vi "rsscope_core_global.vi"() -> ()   [LabVIEW 2018] (continued)
MIL1553 trigger word count/ mode code settings."}, {"Level"=5, "Class Only"=FALSE, "Identifier"="RSSCOPE_ATTR_PROTOCOL_MIL1553_TRIGGER_WORD_COUNT_PATTERN_CONDITION", "Descriptive Name"="Protocol MIL1553 Trigger Word Count Pattern Condition", "Data Type"=0, "Command"="TRIG{Trigger}:MILS:CMD:CCON", "Access"=2, "Range Table"="rsscope_rngProtocolMIL1553WordCountOperator", "Read Callback"="", "Write Callback"="", "Supported Models"="RTO|RTP", "Instrument Options"="", "Flags"=0, "Help"="Sets the operator to set a specific data word count or mode code pattern.\n\nAvailable Repeated Capabilities:\nTrigger: TrigA, TrigB, TrigR\r\n\nRemote-control command(s):\nTRIGger<m>:MILStd:CMD:CCONdition"}, {"Level"=5, "Class Only"=FALSE, "Identifier"="RSSCOPE_ATTR_PROTOCOL_MIL1553_TRIGGER_WORD_COUNT_PATTERN_MIN", "Descriptive Name"="Protocol MIL1553 Trigger Word Count Pattern Min", "Data Type"=2, "Command"="TRIG{Trigger}:MILS:CMD:CMIN", "Access"=2, "Range Table"="", "Read Callback"="", "Write Callback"="", "Supported Models"="RTO|RTP", "Instrument Options"="", "Flags"=0, "Help"="Specifies a data word count/mode code pattern or sets the start value of a pattern range.\n\nAvailable Repeated Capabilities:\nTrigger: TrigA, TrigB, TrigR\r\n\nRemote-control command(s):\nTRIGger<m>:MILStd:CMD:CMIN"}, {"Level"=5, "Class Only"=FALSE, "Identifier"="RSSCOPE_ATTR_PROTOCOL_MIL1553_TRIGGER_WORD_COUNT_PATTERN_MAX", "Descriptive Name"="Protocol MIL1553 Trigger Word Count Pattern Max", "Data Type"=2, "Command"="TRIG{Trigger}:MILS:CMD:CMAX", "Access"=2, "Range Table"="", "Read Callback"="", "Write Callback"="", "Supported Models"="RTO|RTP", "Instrument Options"="", "Flags"=0, "Help"="Sets the end value of a data word count/mode code pattern if &apos;Word Count Condition&apos; is set to InRange or OutOfRange.\n\nAvailable Repeated Capabilities:\nTrigger: TrigA, TrigB, TrigR\r\n\nRemote-control command(s):\nTRIGger<m>:MILStd:CMD:CMAX"}, {"Level"=3, "Class Only"=TRUE, "Identifier"="", "Descriptive Name"="Status Flags", "Data Type"=0, "Command"="", "Access"=0, "Range Table"="", "Read Callback"="", "Write Callback"="", "Supported Models"="", "Instrument Options"="", "Flags"=0, "Help"="Specifies the values of the status flags. You can use the following characters: 1; 0; or X (don&apos;t care)."}, {"Level"=4, "Class Only"=FALSE, "Identifier"="RSSCOPE_ATTR_PROTOCOL_MIL1553_TRIGGER_STATUS_FLAG_MESSAGE_ERROR", "Descriptive Name"="Protocol MIL1553 Trigger Status Flag Message Error", "Data Type"=0, "Command"="TRIG{Trigger}:MILS:STAT:MERR", "Access"=2, "Range Table"="rsscope_rngProtocolMIL1553TriggerStatusFlags", "Read Callback"="", "Write Callback"="", "Supported Models"="RTO|RTP", "Instrument Options"="", "Flags"=0, "Help"="Triggers on the state of the message error bit of the status word if &apos;Trigger Mode&apos; is set to StatusWord.\n\nAvailable Repeated Capabilities:\nTrigger: TrigA, TrigB, TrigR\r\n\nRemote-control command(s):\nTRIGger<m>:MILStd:STATus:MERRor"}, {"Level"=4, "Class Only"=FALSE, "Identifier"="RSSCOPE_ATTR_PROTOCOL_MIL1553_TRIGGER_STATUS_FLAG_BUSY", "Descriptive Name"="Protocol MIL1553 Trigger Status Flag Busy", "Data Type"=0, "Command"="TRIG{Trigger}:MILS:STAT:BUSY", "Access"=2, "Range Table"="rsscope_rngProtocolMIL1553TriggerStatusFlags", "Read Callback"="", "Write Callback"="", "Supported Models"="RTO|RTP", "Instrument Options"="", "Flags"=0, "Help"="Triggers on the state of the busy bit of the status word if &apos;Trigger Mode&apos; is set to StatusWord.\n\nAvailable Repeated Capabilities:\nTrigger: TrigA, TrigB, TrigR\r\n\nRemote-control command(s):\nTRIGger<m>:MILStd:STATus:BUSY"}, {"Level"=4, "Class Only"=FALSE, "Identifier"="RSSCOPE_ATTR_PROTOCOL_MIL1553_TRIGGER_STATUS_FLAG_INSTRUMENTATION", "Descriptive Name"="Protocol MIL1553 Trigger Status Flag Instrumentation", "Data Type"=0, "Command"="TRIG{Trigger}:MILS:STAT:INST", "Access"=2, "Range Table"="rsscope_rngProtocolMIL1553TriggerStatusFlags", "Read Callback"="", "Write Callback"="", "Supported Models"="RTO|RTP", "Instrument Options"="", "Flags"=0, "Help"="Triggers on the state of the instrumentation bit of the status word if &apos;Trigger Mode&apos; is set to StatusWord.\n\nAvailable Repeated Capabilities:\nTrigger: TrigA, TrigB, TrigR\r\n\nRemote-control command(s):\nTRIGger<m>:MILStd:STATus:INSTrument"}, {"Level"=4, "Class Only"=FALSE, "Identifier"="RSSCOPE_ATTR_PROTOCOL_MIL1553_TRIGGER_STATUS_FLAG_SUBSYSTEM", "Descriptive Name"="Protocol MIL1553 Trigger Status Flag Subsystem", "Data Type"=0, "Command"="TRIG{Trigger}:MILS:STAT:SUBS", "Access"=2, "Range Table"="rsscope_rngProtocolMIL1553TriggerStatusFlags", "Read Callback"="", "Write Callback"="", "Supported Models"="RTO|RTP", "Instrument Options"="", "Flags"=0, "Help"="Triggers on the state of the subsystem flag bit of the status word if &apos;Trigger Mode&apos; is set to StatusWord.\n\nAvailable Repeated Capabilities:\nTrigger: TrigA, TrigB, TrigR\r\n\nRemote-control command(s):\nTRIGger<m>:MILStd:STATus:SUBSystem"}, {"Level"=4, "Class Only"=FALSE, "Identifier"="RSSCOPE_ATTR_PROTOCOL_MIL1553_TRIGGER_STATUS_FLAG_SERVICE_REQUEST", "Descriptive Name"="Protocol MIL1553 Trigger Status Flag Service Request", "Data Type"=0, "Command"="TRIG{Trigger}:MILS:STAT:SREQ", "Access"=2, "Range Table"="rsscope_rngProtocolMIL1553TriggerStatusFlags", "Read Callback"="", "Write Callback"="", "Supported Models"="RTO|RTP", "Instrument Options"="", "Flags"=0, "Help"="Triggers on the state of the service request bit of the status word if &apos;Trigger Mode&apos; is set to StatusWord.\n\nAvailable Repeated Capabilities:\nTrigger: TrigA, TrigB, TrigR\r\n\nRemote-control command(s):\nTRIGger<m>:MILStd:STATus:SREQuest"}, {"Level"=4, "Class Only"=FALSE, "Identifier"="RSSCOPE_ATTR_PROTOCOL_MIL1553_TRIGGER_STATUS_FLAG_DYNAMIC_BUS_CONTROL", "Descriptive Name"="Protocol MIL1553 Trigger Status Flag Dynamic Bus Control", "Data Type"=0, "Command"="TRIG{Trigger}:MILS:STAT:DBC", "Access"=2, "Range Table"="rsscope_rngProtocolMIL1553TriggerStatusFlags", "Read Callback"="", "Write Callback"="", "Supported Models"="RTO|RTP", "Instrument Options"="", "Flags"=0, "Help"="Triggers on the state of the dynamic bus control accept bit of the status word if &apos;Trigger Mode&apos; is set to StatusWord.\n\nAvailable Repeated Capabilities:\nTrigger: TrigA, TrigB, TrigR\r\n\nRemote-control command(s):\nTRIGger<m>:MILStd:STATus:DBCaccept"}, {"Level"=4, "Class Only"=FALSE, "Identifier"="RSSCOPE_ATTR_PROTOCOL_MIL1553_TRIGGER_STATUS_FLAG_BROADCAST_COMMAND", "Descriptive Name"="Protocol MIL1553 Trigger Status Flag Broadcast Command", "Data Type"=0, "Command"="TRIG{Trigger}:MILS:STAT:BCR", "Access"=2, "Range Table"="rsscope_rngProtocolMIL1553TriggerStatusFlags", "Read Callback"="", "Write Callback"="", "Supported Models"="RTO|RTP", "Instrument Options"="", "Flags"=0, "Help"="Triggers on the state of the broadcast command received bit of the status word if &apos;Trigger Mode&apos; is set to StatusWord.\n\nAvailable Repeated Capabilities:\nTrigger: TrigA, TrigB, TrigR\r\n\nRemote-control command(s):\nTRIGger<m>:MILStd:STATus:BCReceived"}, {"Level"=4, "Class Only"=FALSE, "Identifier"="RSSCOPE_ATTR_PROTOCOL_MIL1553_TRIGGER_STATUS_FLAG_TERMINAL", "Descriptive Name"="Protocol MIL1553 Trigger Status Flag Terminal", "Data Type"=0, "Command"="TRIG{Trigger}:MILS:STAT:TERM", "Access"=2, "Range Table"="rsscope_rngProtocolMIL1553TriggerStatusFlags", "Read Callback"="", "Write Callback"="", "Supported Models"="RTO|RTP", "Instrument Options"="", "Flags"=0, "Help"="Triggers on the state of the terminal flag bit of the status word if &apos;Trigger Mode&apos; is set to StatusWord.\n\nAvailable Repeated Capabilities:\nTrigger: TrigA, TrigB, TrigR\r\n\nRemote-control command(s):\nTRIGger<m>:MILStd:STATus:TERMinal"}, {"Level"=3, "Class Only"=TRUE, "Identifier"="", "Descriptive Name"="Error Condition", "Data Type"=0, "Command"="", "Access"=0, "Range Table"="", "Read Callback"="", "Write Callback"="", "Supported Models"="", "Instrument Options"="", "Flags"=0, "Help"="Specifies the error conditions to be triggered on."}, {"Level"=4, "Class Only"=FALSE, "Identifier"="RSSCOPE_ATTR_PROTOCOL_MIL1553_TRIGGER_ERROR_SYNCHRONIZATION_ERROR", "Descriptive Name"="Protocol MIL1553 Trigger Error Synchronization Error", "Data Type"=3, "Command"="TRIG{Trigger}:MILS:ERR:SYNC", "Access"=2, "Range Table"="", "Read Callback"="", "Write Callback"="", "Supported Models"="RTO|RTP", "Instrument Options"="", "Flags"=0, "Help"="Triggers on an error of the synchronization.\n\nAvailable Repeated Capabilities:\nTrigger: TrigA, TrigB, TrigR\r\n\nRemote-control command(s):\nTRIGger<m>:MILStd:ERRor:SYNC"}, {"Level"=4, "Class Only"=FALSE, "Identifier"="RSSCOPE_ATTR_PROTOCOL_MIL1553_TRIGGER_ERROR_PARITY_ERROR", "Descriptive Name"="Protocol MIL1553 Trigger Error Parity Error", "Data Type"=3, "Command"="TRIG{Trigger}:MILS:ERR:PAR", "Access"=2, "Range Table"="", "Read Callback"="", "Write Callback"="", "Supported Models"="RTO|RTP", "Instrument Options"="", "Flags"=0, "Help"="Checks the parity of every word and triggers if the parity is even.\n\nAvailable Repeated Capabilities:\nTrigger: TrigA, TrigB, TrigR\r\n\nRemote-control command(s):\nTRIGger<m>:MILStd:ERRor:PARity"}, {"Level"=4, "Class Only"=FALSE, "Identifier"="RSSCOPE_ATTR_PROTOCOL_MIL1553_TRIGGER_ERROR_MANCHESTER_CODING_ERROR", "Descriptive Name"="Protocol MIL1553 Trigger Error Manchester Coding Error", "Data Type"=3, "Command"="TRIG{Trigger}:MILS:ERR:MANC", "Access"=2, "Range Table"="", "Read Callback"="", "Write Callback"="", "Supported Models"="RTO|RTP", "Instrument Options"="", "Flags"=0, "Help"="Triggers if there is an error in the Manchester coding of the signal.\n\nAvailable Repeated Capabilities:\nTrigger: TrigA, TrigB, TrigR\r\n\nRemote-control command(s):\nTRIGger<m>:MILStd:ERRor:MANChester"}, {"Level"=4, "Class Only"=TRUE, "Identifier"="", "Descriptive Name"="Timing", "Data Type"=0, "Command"="", "Access"=0, "Range Table"="", "Read Callback"="", "Write Callback"="", "Supported Models"="", "Instrument Options"="", "Flags"=0, "Help"="Specifies the timeouts to be triggered on."}, {"Level"=5, "Class Only"=FALSE, "Identifier"="RSSCOPE_ATTR_PROTOCOL_MIL1553_TRIGGER_ERROR_TIMING_MIN_GAP_ENABLED", "Descriptive Name"="Protocol MIL1553 Trigger Error Timing Min Gap Enabled", "Data Type"=3, "Command"="TRIG{Trigger}:MILS:MING:SEL", "Access"=2, "Range Table"="", "Read Callback"="", "Write Callback"="", "Supported Models"="RTO|RTP", "Instrument Options"="", "Flags"=0, "Help"="Enables triggering when the minimum gap is out of range.\n\nAvailable Repeated Capabilities:\nTrigger: TrigA, TrigB, TrigR\r\n\nRemote-control command(s):\nTRIGger<m>:MILStd:MINGap:SELect"}, {"Level"=5, "Class Only"=FALSE, "Identifier"="RSSCOPE_ATTR_PROTOCOL_MIL1553_TRIGGER_ERROR_TIMING_MIN_GAP_TIME", "Descriptive Name"="Protocol MIL1553 Trigger Error Timing Min Gap Time", "Data Type"=1, "Command"="TRIG{Trigger}:MILS:MING:BITS", "Access"=2, "Range Table"="rsscope_rngProtocolMIL1553TriggerErrorTimingMinGapTime", "Read Callback"="", "Write Callback"="", "Supported Models"="RTO|RTP", "Instrument Options"="", "Flags"=0, "Help"="Sets the value for the minimum gap to be triggered.\n\nAvailable Repeated Capabilities:\nTrigger: TrigA, TrigB, TrigR\r\n\nRemote-control command(s):\nTRIGger<m>:MILStd:MINGap:BITS"}, {"Level"=5, "Class Only"=FALSE, "Identifier"="RSSCOPE_ATTR_PROTOCOL_MIL1553_TRIGGER_ERROR_TIMING_MAX_RESPONSE_ENABLED", "Descriptive Name"="Protocol MIL1553 Trigger Error Timing Max Response Enabled", "Data Type"=3, "Command"="TRIG{Trigger}:MILS:MAXR:SEL", "Access"=2, "Range Table"="", "Read Callback"="", "Write Callback"="", "Supported Models"="RTO|RTP", "Instrument Options"="", "Flags"=0, "Help"="Enables triggering when the maximum gap is out of range.\n\nAvailable Repeated Capabilities:\nTrigger: TrigA, TrigB, TrigR\r\n\nRemote-control command(s):\nTRIGger<m>:MILStd:MAXResponse:SELect"}, {"Level"=5, "Class Only"=FALSE, "Identifier"="RSSCOPE_ATTR_PROTOCOL_MIL1553_TRIGGER_ERROR_TIMING_MAX_RESPONSE", "Descriptive Name"="Protocol MIL1553 Trigger Error Timing Max Response", "Data Type"=1, "Command"="TRIG{Trigger}:MILS:MAXR:BITS", "Access"=2, "Range Table"="rsscope_rngProtocolMIL1553TriggerErrorTimingMaxResponse", "Read Callback"="", "Write Callback"="", "Supported Models"="RTO|RTP", "Instrument Options"="", "Flags"=0, "Help"="Sets the value for the maximum gap to be triggered.\n\nAvailable Repeated Capabilities:\nTrigger: TrigA, TrigB, TrigR\r\n\nRemote-control command(s):\nTRIGger<m>:MILStd:MAXResponse:BITS"}, {"Level"=2, "Class Only"=TRUE, "Identifier"="", "Descriptive Name"="ARINC 429", "Data Type"=0, "Command"="", "Access"=0, "Range Table"="", "Read Callback"="", "Write Callback"="", "Supported Models"="", "Instrument Options"="", "Flags"=0, "Help"="Configures ARINC 429 trigger settings."}, {"Level"=3, "Class Only"=FALSE, "Identifier"="RSSCOPE_ATTR_PROTOCOL_ARINC429_TRIGGER_MODE", "Descriptive Name"="Protocol ARINC429 Trigger Mode", "Data Type"=0, "Command"="TRIG{Trigger}:ARIN:TYPE", "Access"=2, "Range Table"="rsscope_rngProtocolARINC429TriggerMode", "Read Callback"="", "Write Callback"="", "Supported Models"="RTO|RTP", "Instrument Options"="", "Flags"=0, "Help"="Sets the trigger type for ARINC 429 analysis.\n\nAvailable Repeated Capabilities:\nTrigger: TrigA, TrigB, TrigR\r\n\nRemote-control command(s):\nTRIGger<m>:ARINc:TYPE"}, {"Level"=3, "Class Only"=TRUE, "Identifier"="", "Descriptive Name"="LabelData", "Data Type"=0, "Command"="", "Access"=0, "Range Table"="", "Read Callback"="", "Write Callback"="", "Supported Models"="", "Instrument Options"="", "Flags"=0, "Help"="Configures ARINC 429 trigger label+data settings."}, {"Level"=4, "Class Only"=FALSE, "Identifier"="RSSCOPE_ATTR_PROTOCOL_ARINC429_TRIGGER_LABEL_DATA_SDI", "Descriptive Name"="Protocol ARINC429 Trigger Label Data SDI", "Data Type"=0, "Command"="TRIG{Trigger}:ARIN:SDI", "Access"=2, "Range Table"="", "Read Callback"="rsscope_ConvertFromBinary_ReadCallback.vi", "Write Callback"="", "Supported Models"="RTO|RTP", "Instrument Options"="", "Flags"=0, "Help"="Sets the source/destination identifier (SDI) bits.\n\nAvailable Repeated Capabilities:\nTrigger: TrigA, TrigB, TrigR\r\n\nRemote-control command(s):\nTRIGger<m>:ARINc:SDI"}, {"Level"=4, "Class Only"=FALSE, "Identifier"="RSSCOPE_ATTR_PROTOCOL_ARINC429_TRIGGER_LABEL_DATA_SSM", "Descriptive Name"="Protocol ARINC429 Trigger Label Data SSM", "Data Type"=0, "Command"="TRIG{Trigger}:ARIN:SSM", "Access"=2, "Range Table"="", "Read Callback"="rsscope_ConvertFromBinary_ReadCallback.vi", "Write Callback"="", "Supported Models"="RTO|RTP", "Instrument Options"="", "Flags"=0, "Help"="Sets the sign/status matrix (SSM) bits.\n\nAvailable Repeated Capabilities:\nTrigger: TrigA, TrigB, TrigR\r\n\nRemote-control command(s):\nTRIGger<m>:ARINc:SSM"}, {"Level"=4, "Class Only"=FALSE, "Identifier"="RSSCOPE_ATTR_PROTOCOL_ARINC429_TRIGGER_LABEL_PATTERN_CONDITION", "Descriptive Name"="Protocol ARINC429 Trigger Label Pattern Condition", "Data Type"=0, "Command"="TRIG{Trigger}:ARIN:LAB:COND", "Access"=2, "Range Table"="rsscope_rngProtocolARINC429LabelOperator", "Read Callback"="", "Write Callback"="", "Supported Models"="RTO|RTP", "Instrument Options"="", "Flags"=0, "Help"="Sets the condition for the label. You can define an exact label or a label range.\n\nAvailable Repeated Capabilities:\nTrigger: TrigA, TrigB, TrigR\r\n\nRemote-control command(s):\nTRIGger<m>:ARINc:LABel:CONDition"}, {"Level"=4, "Class Only"=FALSE, "Identifier"="RSSCOPE_ATTR_PROTOCOL_ARINC429_TRIGGER_LABEL_PATTERN_MIN", "Descriptive Name"="Protocol ARINC429 Trigger Label Pattern Min", "Data Type"=2, "Command"="TRIG{Trigger}:ARIN:LAB:MIN", "Access"=2, "Range Table"="", "Read Callback"="", "Write Callback"="", "Supported Models"="RTO|RTP", "Instrument Options"="", "Flags"=0, "Help"="Defines the minimum bit pattern for the label.\n\nAvailable Repeated Capabilities:\nTrigger: TrigA, TrigB, TrigR\r\n\nRemote-control command(s):\nTRIGger<m>:ARINc:LABel:MIN"}, {"Level"=4, "Class Only"=FALSE, "Identifier"="RSSCOPE_ATTR_PROTOCOL_ARINC429_TRIGGER_LABEL_PATTERN_MAX", "Descriptive Name"="Protocol ARINC429 Trigger Label Pattern Max", "Data Type"=2, "Command"="TRIG{Trigger}:ARIN:LAB:MAX", "Access"=2, "Range Table"="", "Read Callback"="", "Write Callback"="", "Supported Models"="RTO|RTP", "Instrument Options"="", "Flags"=0, "Help"="Sets the end value of a label pattern if &apos;Label Pattern Condition&apos; is set to InRange or OutOfRange.\n\nAvailable Repeated Capabilities:\nTrigger: TrigA, TrigB, TrigR\r\n\nRemote-control command(s):\nTRIGger<m>:ARINc:LABel:MAX"}, {"Level"=4, "Class Only"=FALSE, "Identifier"="RSSCOPE_ATTR_PROTOCOL_ARINC429_TRIGGER_DATA_PATTERN_CONDITION", "Descriptive Name"="Protocol ARINC429 Trigger Data Pattern Condition", "Data Type"=0, "Command"="TRIG{Trigger}:ARIN:DATA:COND", "Access"=2, "Range Table"="rsscope_rngProtocolARINC429DataOperator", "Read Callback"="", "Write Callback"="", "Supported Models"="RTO|RTP", "Instrument Options"="", "Flags"=0, "Help"="Sets the condition for the data. You can define an exact data patterm or a data range.\n\nAvailable Repeated Capabilities:\nTrigger: TrigA, TrigB, TrigR\r\n\nRemote-control command(s):\nTRIGger<m>:ARINc:DATA:CONDition"}, {"Level"=4, "Class Only"=FALSE, "Identifier"="RSSCOPE_ATTR_PROTOCOL_ARINC429_TRIGGER_DATA_PATTERN_MIN", "Descriptive Name"="Protocol ARINC429 Trigger Data Pattern Min", "Data Type"=2, "Command"="TRIG{Trigger}:ARIN:DATA:MIN", "Access"=2, "Range Table"="", "Read Callback"="", "Write Callback"="", "Supported Models"="RTO|RTP", "Instrument Options"="", "Flags"=0, "Help"="Defines the minimum bit pattern for the data.\n\nAvailable Repeated Capabilities:\nTrigger: TrigA, TrigB, TrigR\r\n\nRemote-control command(s):\nTRIGger<m>:ARINc:DATA:MIN"}, {"Level"=4, "Class Only"=FALSE, "Identifier"="RSSCOPE_ATTR_PROTOCOL_ARINC429_TRIGGER_DATA_PATTERN_MAX", "Descriptive Name"="Protocol ARINC429 Trigger Data Pattern Max", "Data Type"=2, "Command"="TRIG{Trigger}:ARIN:DATA:MAX", "Access"=2, "Range Table"="", "Read Callback"="", "Write Callback"="", "Supported Models"="RTO|RTP", "Instrument Options"="", "Flags"=0, "Help"="Sets the end value of a data pattern if &apos;Data Pattern Condition&apos; is set to InRange or OutOfRange.\n\nAvailable Repeated Capabilities:\nTrigger: TrigA, TrigB, TrigR\r\n\nRemote-control command(s):\nTRIGger<m>:ARINc:DATA:MAX"}, {"Level"=3, "Class Only"=TRUE, "Identifier"="", "Descriptive Name"="Error Condition", "Data Type"=0, "Command"="", "Access"=0, "Range Table"="", "Read Callback"="", "Write Callback"="", "Supported Models"="", "Instrument Options"="", "Flags"=0, "Help"="Specifies the error conditions to be triggered on."}, {"Level"=4, "Class Only"=FALSE, "Identifier"="RSSCOPE_ATTR_PROTOCOL_ARINC429_TRIGGER_ERROR_CODING_ERROR", "Descriptive Name"="Protocol ARINC429 Trigger Error Coding Error", "Data Type"=3, "Command"="TRIG{Trigger}:ARIN:ERR:COD", "Access"=2, "Range Table"="", "Read Callback"="", "Write Callback"="", "Supported Models"="RTO|RTP", "Instrument Options"="", "Flags"=0, "Help"="Enables triggering when a coding error occurs.\n\nAvailable Repeated Capabilities:\nTrigger: TrigA, TrigB, TrigR\r\n\nRemote-control command(s):\nTRIGger<m>:ARINc:ERRor:CODing"}, {"Level"=4, "Class Only"=FALSE, "Identifier"="RSSCOPE_ATTR_PROTOCOL_ARINC429_TRIGGER_ERROR_PARITY_ERROR", "Descriptive Name"="Protocol ARINC429 Trigger Error Parity Error", "Data Type"=3, "Command"="TRIG{Trigger}:ARIN:ERR:PAR", "Access"=2, "Range Table"="", "Read Callback"="", "Write Callback"="", "Supported Models"="RTO|RTP", "Instrument Options"="", "Flags"=0, "Help"="Enables triggering when a parity error occurs.\n\nAvailable Repeated Capabilities:\nTrigger: TrigA, TrigB, TrigR\r\n\nRemote-control command(s):\nTRIGger<m>:ARINc:ERRor:PARity"}, {"Level"=4, "Class Only"=TRUE, "Identifier"="", "Descriptive Name"="Timing", "Data Type"=0, "Command"="", "Access"=0, "Range Table"="", "Read Callback"="", "Write Callback"="", "Supported Models"="", "Instrument Options"="", "Flags"=0, "Help"="Specifies the timeouts to be triggered on."}, {"Level"=5, "Class Only"=FALSE, "Identifier"="RSSCOPE_ATTR_PROTOCOL_ARINC429_TRIGGER_ERROR_TIMING_MIN_GAP_ENABLED", "Descriptive Name"="Protocol ARINC429 Trigger Error Timing Min Gap Enabled", "Data Type"=3, "Command"="TRIG{Trigger}:ARIN:MING:SEL", "Access"=2, "Range Table"="", "Read Callback"="", "Write Callback"="", "Supported Models"="RTO|RTP", "Instrument Options"="", "Flags"=0, "Help"="Enables triggering when the minimum gap is out of range.\n\nAvailable Repeated Capabilities:\nTrigger: TrigA, TrigB, TrigR\r\n\nRemote-control command(s):\nTRIGger<m>:ARINc:MINGap:SELect"}, {"Level"=5, "Class Only"=FALSE, "Identifier"="RSSCOPE_ATTR_PROTOCOL_ARINC429_TRIGGER_ERROR_TIMING_MIN_GAP_BITS", "Descriptive Name"="Protocol ARINC429 Trigger Error Timing Min Gap Bits", "Data Type"=0, "Command"="TRIG{Trigger}:ARIN:MING:BITS", "Access"=2, "Range Table"="rsscope_rngProtocolARINC429TriggerErrorTimingMinGapBits", "Read Callback"="", "Write Callback"="", "Supported Models"="RTO|RTP", "Instrument Options"="", "Flags"=0, "Help"="Sets the value for the minimum gap to be triggered on.\n\nAvailable Repeated Capabilities:\nTrigger: TrigA, TrigB, TrigR\r\n\nRemote-control command(s):\nTRIGger<m>:ARINc:MINGap:BITS"}, {"Level"=5, "Class Only"=FALSE, "Identifier"="RSSCOPE_ATTR_PROTOCOL_ARINC429_TRIGGER_ERROR_TIMING_MAX_GAP_ENABLED", "Descriptive Name"="Protocol ARINC429 Trigger Error Timing Max Gap Enabled", "Data Type"=3, "Command"="TRIG{Trigger}:ARIN:MAXG:SEL", "Access"=2, "Range Table"="", "Read Callback"="", "Write Callback"="", "Supported Models"="RTO|RTP", "Instrument Options"="", "Flags"=0, "Help"="Enables triggering when the maximum gap is out of range.\n\nAvailable Repeated Capabilities:\nTrigger: TrigA, TrigB, TrigR\r\n\nRemote-control command(s):\nTRIGger<m>:ARINc:MAXGap:SELect"}, {"Level"=5, "Class Only"=FALSE, "Identifier"="RSSCOPE_ATTR_PROTOCOL_ARINC429_TRIGGER_ERROR_TIMING_MAX_GAP_BITS", "Descriptive Name"="Protocol ARINC429 Trigger Error Timing Max Gap Bits", "Data Type"=0, "Command"="TRIG{Trigger}:ARIN:MAXG:BITS", "Access"=2, "Range Table"="rsscope_rngProtocolARINC429TriggerErrorTimingMaxGapBits", "Read Callback"="", "Write Callback"="", "Supported Models"="RTO|RTP", "Instrument Options"="", "Flags"=0, "Help"="Sets the value for the maximum gap to be triggered on.\n\nAvailable Repeated Capabilities:\nTrigger: TrigA, TrigB, TrigR\r\n\nRemote-control command(s):\nTRIGger<m>:ARINc:MAXGap:BITS"}, {"Level"=2, "Class Only"=TRUE, "Identifier"="", "Descriptive Name"="RFFE", "Data Type"=0, "Command"="", "Access"=0, "Range Table"="", "Read Callback"="", "Write Callback"="", "Supported Models"="", "Instrument Options"="", "Flags"=0, "Help"="Configures RFFE trigger settings."}, {"Level"=3, "Class Only"=FALSE, "Identifier"="RSSCOPE_ATTR_PROTOCOL_RFFE_TRIGGER_TYPE", "Descriptive Name"="Protocol RFFE Trigger Type", "Data Type"=0, "Command"="TRIG{Trigger}:RFFE:TYPE", "Access"=2, "Range Table"="rsscope_rngProtocolRFFETriggerType", "Read Callback"="", "Write Callback"="", "Supported Models"="", "Instrument Options"="K40", "Flags"=0, "Help"="Configures the trigger type for RFFE analysis.\n\nAvailable Repeated Capabilities:\nTrigger: TrigA, TrigB, TrigR\r\n\nRemote-control command(s):\nTRIGger<m>:RFFE:TYPE"}, {"Level"=3, "Class Only"=FALSE, "Identifier"="RSSCOPE_ATTR_PROTOCOL_RFFE_TRIGGER_INTERRUPT_PATTERN", "Descriptive Name"="Protocol RFFE Trigger Interrupt Pattern", "Data Type"=2, "Command"="TRIG{Trigger}:RFFE:INT", "Access"=2, "Range Table"="", "Read Callback"="", "Write Callback"="", "Supported Models"="", "Instrument Options"="", "Flags"=0, "Help"="Sets the interrupt pattern for the interupt summary and notification trigger type.\n\nAvailable Repeated Capabilities:\nTrigger: TrigA, TrigB, TrigR\r\n\nRemote-control command(s):\nTRIGger<m>:RFFE:INTerrupt"}, {"Level"=3, "Class Only"=TRUE, "Identifier"="", "Descriptive Name"="Slave Address", "Data Type"=0, "Command"="", "Access"=0, "Range Table"="", "Read Callback"="", "Write Callback"="", "Supported Models"="", "Instrument Options"="", "Flags"=0, "Help"="Defines the addess of the slave. The slave address setup consists of the condition and one or two address patterns"}, {"Level"=4, "Class Only"=FALSE, "Identifier"="RSSCOPE_ATTR_PROTOCOL_RFFE_TRIGGER_SLAVE_CONDITION", "Descriptive Name"="Protocol RFFE Trigger Slave Condition", "Data Type"=0, "Command"="TRIG{Trigger}:RFFE:SADD:COND", "Access"=2, "Range Table"="rsscope_rngProtocolTriggerCondition", "Read Callback"="", "Write Callback"="", "Supported Models"="", "Instrument Options"="K40", "Flags"=0, "Help"="Sets the operator to trigger on a specific pattern or a range.\n\nAvailable Repeated Capabilities:\nTrigger: TrigA, TrigB, TrigR\r\n\nRemote-control command(s):\nTRIGger<m>:RFFE:SADD:CONDition"}, {"Level"=4, "Class Only"=FALSE, "Identifier"="RSSCOPE_ATTR_PROTOCOL_RFFE_TRIGGER_SLAVE_MIN", "Descriptive Name"="Protocol RFFE Trigger Slave Min", "Data Type"=2, "Command"="TRIG{Trigger}:RFFE:SADD:MIN", "Access"=2, "Range Table"="", "Read Callback"="", "Write Callback"="", "Supported Models"="", "Instrument Options"="K40", "Flags"=0, "Help"="Specifies a pattern, or sets the start value of a pattern range.\n\nAvailable Repeated Capabilities:\nTrigger: TrigA, TrigB, TrigR\r\n\nRemote-control command(s):\nTRIGger<m>:RFFE:SADD:MIN"}, {"Level"=4, "Class Only"=FALSE, "Identifier"="RSSCOPE_ATTR_PROTOCOL_RFFE_TRIGGER_SLAVE_MAX", "Descriptive Name"="Protocol RFFE Trigger Slave Max", "Data Type"=2, "Command"="TRIG{Trigger}:RFFE:SADD:MAX", "Access"=2, "Range Table"="", "Read Callback"="", "Write Callback"="", "Supported Models"="", "Instrument Options"="K40", "Flags"=0, "Help"="Sets the end value of an range if the corresponding condition is set to In Range or Out Of Range.\n\nAvailable Repeated Capabilities:\nTrigger: TrigA, TrigB, TrigR\r\n\nRemote-control command(s):\nTRIGger<m>:RFFE:SADD:MAX"}, {"Level"=3, "Class Only"=TRUE, "Identifier"="", "Descriptive Name"="Address", "Data Type"=0, "Command"="", "Access"=0, "Range Table"="", "Read Callback"="", "Write Callback"="", "Supported Models"="", "Instrument Options"="", "Flags"=0, "Help"="Defines the register address. The register address setup consists of the condition and one or two address patterns."}, {"Level"=4, "Class Only"=FALSE, "Identifier"="RSSCOPE_ATTR_PROTOCOL_RFFE_TRIGGER_ADDRESS_CONDITION", "Descriptive Name"="Protocol RFFE Trigger Address Condition", "Data Type"=0, "Command"="TRIG{Trigger}:RFFE:ADDR:COND", "Access"=2, "Range Table"="rsscope_rngProtocolTriggerCondition", "Read Callback"="", "Write Callback"="", "Supported Models"="", "Instrument Options"="K40", "Flags"=0, "Help"="Sets the operator to trigger on a specific pattern or a range.\n\nAvailable Repeated Capabilities:\nTrigger: TrigA, TrigB, TrigR\r\n\nRemote-control command(s):\nTRIGger<m>:RFFE:ADDRess:CONDition"}, {"Level"=4, "Class Only"=FALSE, "Identifier"="RSSCOPE_ATTR_PROTOCOL_RFFE_TRIGGER_ADDRESS_MIN", "Descriptive Name"="Protocol RFFE Trigger Address Min", "Data Type"=2, "Command"="TRIG{Trigger}:RFFE:ADDR:MIN", "Access"=2, "Range Table"="", "Read Callback"="", "Write Callback"="", "Supported Models"="", "Instrument Options"="K40", "Flags"=0, "Help"="Specifies a pattern, or sets the start value of a pattern range.\n\nAvailable Repeated Capabilities:\nTrigger: TrigA, TrigB, TrigR\r\n\nRemote-control command(s):\nTRIGger<m>:RFFE:ADDRess:MIN"}, {"Level"=4, "Class Only"=FALSE, "Identifier"="RSSCOPE_ATTR_PROTOCOL_RFFE_TRIGGER_ADDRESS_MAX", "Descriptive Name"="Protocol RFFE Trigger Address Max", "Data Type"=2, "Command"="TRIG{Trigger}:RFFE:ADDR:MAX", "Access"=2, "Range Table"="", "Read Callback"="", "Write Callback"="", "Supported Models"="", "Instrument Options"="K40", "Flags"=0, "Help"="Sets the end value of an range if the corresponding condition is set to In Range or Out Of Range.\n\nAvailable Repeated Capabilities:\nTrigger: TrigA, TrigB, TrigR\r\n\nRemote-control command(s):\nTRIGger<m>:RFFE:ADDRess:MAX"}, {"Level"=3, "Class Only"=TRUE, "Identifier"="", "Descriptive Name"="Byte Count", "Data Type"=0, "Command"="", "Access"=0, "Range Table"="", "Read Callback"="", "Write Callback"="", "Supported Models"="", "Instrument Options"="", "Flags"=0, "Help"="Defines the number of data frames to be read or written in the command sequence. The setting is available for all &apos;Extended Register&apos; command sequences, which can transfer more than one data frame."}, {"Level"=4, "Class Only"=FALSE, "Identifier"="RSSCOPE_ATTR_PROTOCOL_RFFE_TRIGGER_BYTE_COUNT_CONDITION", "Descriptive Name"="Protocol RFFE Trigger Byte Count Condition", "Data Type"=0, "Command"="TRIG{Trigger}:RFFE:BCO:COND", "Access"=2, "Range Table"="rsscope_rngProtocolTriggerCondition", "Read Callback"="", "Write Callback"="", "Supported Models"="", "Instrument Options"="K40", "Flags"=0, "Help"="Sets the operator to trigger on a specific pattern or a range.\n\nAvailable Repeated Capabilities:\nTrigger: TrigA, TrigB, TrigR\r\n\nRemote-control command(s):\nTRIGger<m>:RFFE:BCOunt:CONDition"}, {"Level"=4, "Class Only"=FALSE, "Identifier"="RSSCOPE_ATTR_PROTOCOL_RFFE_TRIGGER_BYTE_COUNT_MIN", "Descriptive Name"="Protocol RFFE Trigger Byte Count Min", "Data Type"=2, "Command"="TRIG{Trigger}:RFFE:BCO:MIN", "Access"=2, "Range Table"="", "Read Callback"="", "Write Callback"="", "Supported Models"="", "Instrument Options"="K40", "Flags"=0, "Help"="Specifies a pattern, or sets the start value of a pattern range.\n\nAvailable Repeated Capabilities:\nTrigger: TrigA, TrigB, TrigR\r\n\nRemote-control command(s):\nTRIGger<m>:RFFE:BCOunt:MIN"}, {"Level"=4, "Class Only"=FALSE, "Identifier"="RSSCOPE_ATTR_PROTOCOL_RFFE_TRIGGER_BYTE_COUNT_MAX", "Descriptive Name"="Protocol RFFE Trigger Byte Count Max", "Data Type"=2, "Command"="TRIG{Trigger}:RFFE:BCO:MAX", "Access"=2, "Range Table"="", "Read Callback"="", "Write Callback"="", "Supported Models"="", "Instrument Options"="K40", "Flags"=0, "Help"="Sets the end value of an range if the corresponding condition is set to In Range or Out Of Range.\n\nAvailable Repeated Capabilities:\nTrigger: TrigA, TrigB, TrigR\r\n\nRemote-control command(s):\nTRIGger<m>:RFFE:BCOunt:MAX"}, {"Level"=3, "Class Only"=TRUE, "Identifier"="", "Descriptive Name"="Data", "Data Type"=0, "Command"="", "Access"=0, "Range Table"="", "Read Callback"="", "Write Callback"="", "Supported Models"="", "Instrument Options"="", "Flags"=0, "Help"="Defines the data trigger condition. The data setup consists of the condition and one or two data patterns."}, {"Level"=4, "Class Only"=FALSE, "Identifier"="RSSCOPE_ATTR_PROTOCOL_RFFE_TRIGGER_DATA_CONDITION", "Descriptive Name"="Protocol RFFE Trigger Data Condition", "Data Type"=0, "Command"="TRIG{Trigger}:RFFE:DATA:DCON", "Access"=2, "Range Table"="rsscope_rngProtocolTriggerCondition", "Read Callback"="", "Write Callback"="", "Supported Models"="", "Instrument Options"="K40", "Flags"=0, "Help"="Sets the operator to trigger on a specific pattern or a range.\n\nAvailable Repeated Capabilities:\nTrigger: TrigA, TrigB, TrigR\r\n\nRemote-control command(s):\nTRIGger<m>:RFFE:DATA:DCON"}, {"Level"=4, "Class Only"=FALSE, "Identifier"="RSSCOPE_ATTR_PROTOCOL_RFFE_TRIGGER_DATA_MIN", "Descriptive Name"="Protocol RFFE Trigger Data Min", "Data Type"=2, "Command"="TRIG{Trigger}:RFFE:DATA:DMIN", "Access"=2, "Range Table"="", "Read Callback"="", "Write Callback"="", "Supported Models"="", "Instrument Options"="K40", "Flags"=0, "Help"="Specifies a pattern, or sets the start value of a pattern range.\n\nAvailable Repeated Capabilities:\nTrigger: TrigA, TrigB, TrigR\r\n\nRemote-control command(s):\nTRIGger<m>:RFFE:DATA:DMIN"}, {"Level"=4, "Class Only"=FALSE, "Identifier"="RSSCOPE_ATTR_PROTOCOL_RFFE_TRIGGER_DATA_MAX", "Descriptive Name"="Protocol RFFE Trigger Data Max", "Data Type"=2, "Command"="TRIG{Trigger}:RFFE:DATA:DMAX", "Access"=2, "Range Table"="", "Read Callback"="", "Write Callback"="", "Supported Models"="", "Instrument Options"="K40", "Flags"=0, "Help"="Sets the end value of an range if the corresponding condition is set to In Range or Out Of Range.\n\nAvailable Repeated Capabilities:\nTrigger: TrigA, TrigB, TrigR\r\n\nRemote-control command(s):\nTRIGger<m>:RFFE:DATA:DMAX"}, {"Level"=3, "Class Only"=TRUE, "Identifier"="", "Descriptive Name"="Index", "Data Type"=0, "Command"="", "Access"=0, "Range Table"="", "Read Callback"="", "Write Callback"="", "Supported Models"="", "Instrument Options"="", "Flags"=0, "Help"="Defines the data trigger condition. The data setup consists of the condition and one or two data patterns."}, {"Level"=4, "Class Only"=FALSE, "Identifier"="RSSCOPE_ATTR_PROTOCOL_RFFE_TRIGGER_INDEX_CONDITION", "Descriptive Name"="Protocol RFFE Trigger Index Condition", "Data Type"=0, "Command"="TRIG{Trigger}:RFFE:DATA:ICON", "Access"=2, "Range Table"="rsscope_rngProtocolIndexCondition", "Read Callback"="", "Write Callback"="", "Supported Models"="", "Instrument Options"="K40", "Flags"=0, "Help"="Sets the operator to trigger on a specific pattern or a range.\n\nAvailable Repeated Capabilities:\nTrigger: TrigA, TrigB, TrigR\r\n\nRemote-control command(s):\nTRIGger<m>:RFFE:DATA:ICONdition"}, {"Level"=4, "Class Only"=FALSE, "Identifier"="RSSCOPE_ATTR_PROTOCOL_RFFE_TRIGGER_INDEX_MIN", "Descriptive Name"="Protocol RFFE Trigger Index Min", "Data Type"=0, "Command"="TRIG{Trigger}:RFFE:DATA:IMIN", "Access"=2, "Range Table"="", "Read Callback"="", "Write Callback"="", "Supported Models"="", "Instrument Options"="K40", "Flags"=0, "Help"="Specifies a pattern, or sets the start value of a pattern range.\n\nAvailable Repeated Capabilities:\nTrigger: TrigA, TrigB, TrigR\r\n\nRemote-control command(s):\nTRIGger<m>:RFFE:DATA:IMIN"}, {"Level"=4, "Class Only"=FALSE, "Identifier"="RSSCOPE_ATTR_PROTOCOL_RFFE_TRIGGER_INDEX_MAX", "Descriptive Name"="Protocol RFFE Trigger Index Max", "Data Type"=0, "Command"="TRIG{Trigger}:RFFE:DATA:IMAX", "Access"=2, "Range Table"="", "Read Callback"="", "Write Callback"="", "Supported Models"="", "Instrument Options"="K40", "Flags"=0, "Help"="Sets the end value of an range if the corresponding condition is set to In Range or Out Of Range.\n\nAvailable Repeated Capabilities:\nTrigger: TrigA, TrigB, TrigR\r\n\nRemote-control command(s):\nTRIGger<m>:RFFE:DATA:IMAX"}, {"Level"=3, "Class Only"=TRUE, "Identifier"="", "Descriptive Name"="Mask", "Data Type"=0, "Command"="", "Access"=0, "Range Table"="", "Read Callback"="", "Write Callback"="", "Supported Models"="", "Instrument Options"="", "Flags"=0, "Help"="Defines the data trigger condition. The data setup consists of the condition and one or two data patterns."}, {"Level"=4, "Class Only"=FALSE, "Identifier"="RSSCOPE_ATTR_PROTOCOL_RFFE_TRIGGER_MASK_CONDITION", "Descriptive Name"="Protocol RFFE Trigger Mask Condition", "Data Type"=0, "Command"="TRIG{Trigger}:RFFE:MASK:COND", "Access"=2, "Range Table"="RsScope_rngProtocolRFFETriggerMaskCondition", "Read Callback"="", "Write Callback"="", "Supported Models"="", "Instrument Options"="K40", "Flags"=0, "Help"="Sets the operator to trigger on a mask pattern or a range.\n\nAvailable Repeated Capabilities:\nTrigger: TrigA, TrigB, TrigR\r\n\nRemote-control command(s):\nTRIGger<m>:RFFE:MASK:CONDition"}, {"Level"=4, "Class Only"=FALSE, "Identifier"="RSSCOPE_ATTR_PROTOCOL_RFFE_TRIGGER_MASK_MIN", "Descriptive Name"="Protocol RFFE Trigger Mask Min", "Data Type"=2, "Command"="TRIG{Trigger}:RFFE:MASK:MIN", "Access"=2, "Range Table"="", "Read Callback"="", "Write Callback"="", "Supported Models"="", "Instrument Options"="K40", "Flags"=0, "Help"="Specifies a mask pattern, or sets the start value of a mask pattern range.\n\nAvailable Repeated Capabilities:\nTrigger: TrigA, TrigB, TrigR\r\n\nRemote-control command(s):\nTRIGger<m>:RFFE:MASK:MIN"}, {"Level"=4, "Class Only"=FALSE, "Identifier"="RSSCOPE_ATTR_PROTOCOL_RFFE_TRIGGER_MASK_MAX", "Descriptive Name"="Protocol RFFE Trigger Mask Max", "Data Type"=2, "Command"="TRIG{Trigger}:RFFE:MASK:MAX", "Access"=2, "Range Table"="", "Read Callback"="", "Write Callback"="", "Supported Models"="", "Instrument Options"="K40", "Flags"=0, "Help"="Sets the end value of an range if the mask condition is set to In Range or Out Of Range.\n\nAvailable Repeated Capabilities:\nTrigger: TrigA, TrigB, TrigR\r\n\nRemote-control command(s):\nTRIGger<m>:RFFE:MASK:MAX"}, {"Level"=3, "Class Only"=TRUE, "Identifier"="", "Descriptive Name"="Error Conditions", "Data Type"=0, "Command"="", "Access"=0, "Range Table"="", "Read Callback"="", "Write Callback"="", "Supported Models"="", "Instrument Options"="", "Flags"=0, "Help"="This class configures conditions for Error trigger."}, {"Level"=4, "Class Only"=FALSE, "Identifier"="RSSCOPE_ATTR_PROTOCOL_RFFE_TRIGGER_ERROR_SCC", "Descriptive Name"="Protocol RFFE Trigger Error SCC", "Data Type"=3, "Command"="TRIG{Trigger}:RFFE:ERR:SSC", "Access"=2, "Range Table"="", "Read Callback"="", "Write Callback"="", "Supported Models"="", "Instrument Options"="K40", "Flags"=0, "Help"="Enables the trigger on an SSC error - when no valid SSC sequence has been found after the idle time.\n\nAvailable Repeated Capabilities:\nTrigger: TrigA, TrigB, TrigR\r\n\nRemote-control command(s):\nTRIGger<m>:RFFE:ERRor:SSC"}, {"Level"=4, "Class Only"=FALSE, "Identifier"="RSSCOPE_ATTR_PROTOCOL_RFFE_TRIGGER_ERROR_LENGTH", "Descriptive Name"="Protocol RFFE Trigger Error Length", "Data Type"=3, "Command"="TRIG{Trigger}:RFFE:ERR:LENG", "Access"=2, "Range Table"="", "Read Callback"="", "Write Callback"="", "Supported Models"="", "Instrument Options"="K40", "Flags"=0, "Help"="Enables the trigger on a length error - when an incorrect length of the command sequence has been found.\n\nAvailable Repeated Capabilities:\nTrigger: TrigA, TrigB, TrigR\r\n\nRemote-control command(s):\nTRIGger<m>:RFFE:ERRor:LENGth"}, {"Level"=4, "Class Only"=FALSE, "Identifier"="RSSCOPE_ATTR_PROTOCOL_RFFE_TRIGGER_ERROR_BUS_PARK", "Descriptive Name"="Protocol RFFE Trigger Error Bus Park", "Data Type"=3, "Command"="TRIG{Trigger}:RFFE:ERR:BP", "Access"=2, "Range Table"="", "Read Callback"="", "Write Callback"="", "Supported Models"="", "Instrument Options"="K40", "Flags"=0, "Help"="Enables the trigger on a bus park error - when an incorrect bus parlk cycle has been found.\n\nAvailable Repeated Capabilities:\nTrigger: TrigA, TrigB, TrigR\r\n\nRemote-control command(s):\nTRIGger<m>:RFFE:ERRor:BP"}, {"Level"=4, "Class Only"=FALSE, "Identifier"="RSSCOPE_ATTR_PROTOCOL_RFFE_TRIGGER_ERROR_PARITY", "Descriptive Name"="Protocol RFFE Trigger Error Parity", "Data Type"=3, "Command"="TRIG{Trigger}:RFFE:ERR:PAR", "Access"=2, "Range Table"="", "Read Callback"="", "Write Callback"="", "Supported Models"="", "Instrument Options"="K40", "Flags"=0, "Help"="Enables the trigger on incorrect parity bits.\n\nAvailable Repeated Capabilities:\nTrigger: TrigA, TrigB, TrigR\r\n\nRemote-control command(s):\nTRIGger<m>:RFFE:ERRor:PARity"}, {"Level"=4, "Class Only"=FALSE, "Identifier"="RSSCOPE_ATTR_PROTOCOL_RFFE_TRIGGER_ERROR_NO_RESPONSE", "Descriptive Name"="Protocol RFFE Trigger Error No Response", "Data Type"=3, "Command"="TRIG{Trigger}:RFFE:ERR:NOR", "Access"=2, "Range Table"="", "Read Callback"="", "Write Callback"="", "Supported Models"="", "Instrument Options"="K40", "Flags"=0, "Help"="Enables the trigger on any No Response Frame.\n\nAvailable Repeated Capabilities:\nTrigger: TrigA, TrigB, TrigR\r\n\nRemote-control command(s):\nTRIGger<m>:RFFE:ERRor:NOResponse"}, {"Level"=4, "Class Only"=FALSE, "Identifier"="RSSCOPE_ATTR_PROTOCOL_RFFE_TRIGGER_ERROR_UNKNOWN", "Descriptive Name"="Protocol RFFE Trigger Error Unknown", "Data Type"=3, "Command"="TRIG{Trigger}:RFFE:ERR:USEQ", "Access"=2, "Range Table"="", "Read Callback"="", "Write Callback"="", "Supported Models"="", "Instrument Options"="K40", "Flags"=0, "Help"="Enables the trigger on an unknown sequence - when the instrument cannot detect any supported command sequence.\n\nAvailable Repeated Capabilities:\nTrigger: 
